vi "GetActiveDevs.vi"(6 "Legacy (f)?":bool, 8 "error in (no error)":errorcluster) -> (0 "error out":errorcluster, 2 "Active Device Names":string[](array[string]))   [LabVIEW 2011]
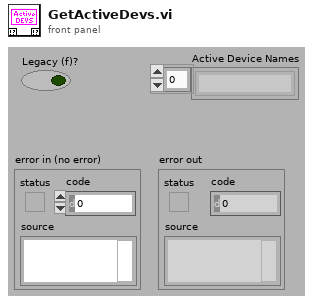
[diagram p1: front panel]
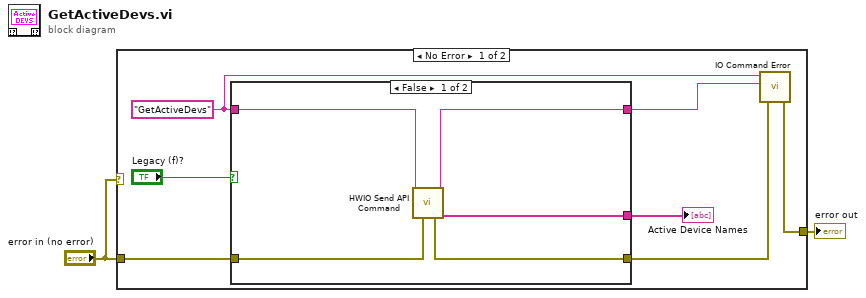
[diagram p0: block diagram]
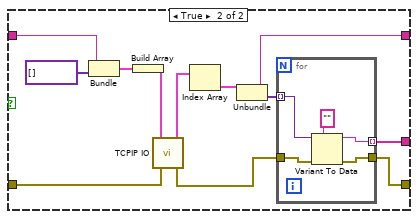
[diagram p2: hidden frame]
diagram:
  n1 = case shown="No Error" "error in (no error)" {
    tunnel: "error in (no error)" -> [w9 w32]
    tunnel: [w7 w32] -> w2
    frame No Error {
      w3 = "GetActiveDevs"
      n2 = case shown="False" "Legacy (f)?" {
        tunnel: w9 -> [w13 w24]
        tunnel: [w14 w22] -> w8
        tunnel: [w11 w21] -> w6
        tunnel: w3 -> [w12 w20]
        tunnel: [w10 w16] -> w5
        frame False {
          n3 = call "HWIO Send API Command.vi"("Action"=w12, "error in (no error)"=w13) -> ("Action out"=w11:string, "error out"=w14:errorcluster, "String out"=w10:string[])  [unwired: 6 in, 5 out]
        }
        frame True {
          n4 = Bundle(w20, "appended array"=variant[] []) -> (w26:cluster{string, "appended array":variant[]})  [unwired: 1 out]
          n5 = Build Array(w26) -> (w17:cluster{string, "appended array":variant[]}[])
          n6 = call "TCPIP IO.vi"("error in (no error)"=w24, "Commands"=w17) -> ("error out"=w23:errorcluster, "Responses"=w19:cluster{string, variant[]}[])  [unwired: 1 in, 3 out]
          n7 = Index Array(array=w19) -> (element=w18:cluster{string, variant[]})  [unwired: 1 in]
          n8 = Unbundle(w18) -> (w21:string, w25:variant[])
          n9 = for {
            tunnel: [w31] -> w22
            tunnel: w23 -> [w30]
            tunnel: w25 -> [w29] mode=indexing
            tunnel: [w28] -> w16 mode=indexing
            n10 = Variant To Data(error in=w30, type="", Variant=w29) -> (data=w28:string, error out=w31:errorcluster)
          }
        }
      }
      "Active Device Names" <- w5
      n11 = call "IO Command Error.vi"("error in (no error)"=w8, "Command Returned (\"\")"=w6, "Command Sent (\"\")"=w3) -> ("error out"=w7:errorcluster)  [unwired: 4 out]
    }
    frame Error {
    }
  }
  "error out" <- w2
